vi "test_F9P.vi"() -> ()   [LabVIEW 2019] (continued)
N,3.578,K,A*10\r\n$GNGGA,064213.00,3723.60796,N,12656.94619,E,1,12,0.68,49.8,M,18.5,M,,*7A\r\n$GNGSA,A,3,17,19,06,05,02,12,09,,,,,,1.13,0.68,0.90,1*00\r\n$GNGSA,A,3,85,70,71,72,,,,,,,,,1.13,0.68,0.90,2*0F\r\n$GNGSA,A,3,36,19,11,04,09,12,,,,,,,1.13,0.68,0.90,3*04\r\n$GNGSA,A,3,28,14,13,11,33,08,10,,,,,,1.13,0.68,0.90,4*04\r\n$GPGSV,4,1,13,02,65,334,34,04,08,037,26,05,48,261,38,06,58,076,46,1*62\r\n$GPGSV,4,2,13,07,06,105,,09,38,057,36,12,18,263,26,13,08,191,,1*6A\r\n$GPGSV,4,3,13,17,19,158,28,19,37,161,30,25,11,294,20,29,07,323,10,1*65\r\n$GPGSV,4,4,13,30,01,134,,1*52\r\n$GPGSV,4,1,13,02,65,334,,04,08,037,19,05,48,261,37,06,58,076,31,6*61\r\n$GPGSV,4,2,13,07,06,105,,09,38,057,33,12,18,263,21,13,08,191,,6*6F\r\n$GPGSV,4,3,13,17,19,158,20,19,37,161,,25,11,294,16,29,07,323,,6*6D\r\n$GPGSV,4,4,13,30,01,134,,6*55\r\n$GLGSV,2,1,06,70,55,030,32,71,68,223,43,72,17,216,27,84,09,133,11,1*73\r\n$GLGSV,2,2,06,85,63,111,32,86,51,337,,1*7B\r\n$GLGSV,2,1,06,70,55,030,,71,68,223,34,72,17,216,20,84,09,133,11,3*77\r\n$GLGSV,2,2,06,85,63,111,25,86,51,337,,3*7F\r\n$GAGSV,3,1,09,02,04,288,08,04,68,087,43,09,44,196,29,11,77,034,39,7*77\r\n$GAGSV,3,2,09,12,32,114,28,18,55,286,44,19,17,042,25,25,01,241,,7*7C\r\n$GAGSV,3,3,09,36,34,314,20,7*4C\r\n$GAGSV,3,1,09,02,04,288,,04,68,087,36,09,44,196,24,11,77,034,26,2*7B\r\n$GAGSV,3,2,09,12,32,114,22,18,55,286,41,19,17,042,23,25,01,241,,2*70\r\n$GAGSV,3,3,09,36,34,314,21,2*48\r\n$GBGSV,4,1,13,04,35,133,,05,09,257,,06,27,182,,07,09,201,,1*7B\r\n$GBGSV,4,2,13,08,65,355,26,09,07,194,,10,16,222,,11,38,142,27,1*71\r\n$GBGSV,4,3,13,13,50,314,19,14,77,038,42,28,58,310,30,33,72,237,42,1*71\r\n$GBGSV,4,4,13,34,13,141,,1*45\r\n$GBGSV,4,1,13,04,35,133,,05,09,257,,06,27,182,,07,09,201,,3*79\r\n$GBGSV,4,2,13,08,65,355,26,09,07,194,,10,16,222,19,11,38,142,29,3*75\r\n$GBGSV,4,3,13,13,50,314,19,14,77,038,38,28,58,310,,33,72,237,,3*7B\r\n$GBGSV,4,4,13,34,13,141,,3*47\r\n$GNGLL,3723.60796,N,12656.94619,E,064213.00,A,A*7B\r\n$GNRMC,064214.00,A,3723.60817,N,12656.94692,E,2.319,73.22,250720,,,A,V*3B\r\n$GNVTG,73.22,T,,M,2.319,N,4.294,K,A*15\r\n$GNGGA,064214.00,3723.60817,N,12656.94692,E,1,12,0.71,49.3,M,18.5,M,,*7B\r\n$GNGSA,A,3,17,19,06,05,02,12,09,,,,,,1.14,0.71,0.90,1*0F\r\n$GNGSA,A,3,85,70,71,72,,,,,,,,,1.14,0.71,0.90,2*00\r\n$GNGSA,A,3,36,19,11,04,09,12,,,,,,,1.14,0.71,0.90,3*0B\r\n$GNGSA,A,3,28,14,13,11,33,08,10,,,,,,1.14,0.71,0.90,4*0B\r\n$GPGSV,4,1,13,02,65,334,29,04,08,037,31,05,48,261,39,06,58,076,39,1*61\r\n$GPGSV,4,2,13,07,06,105,,09,38,057,39,12,18,263,29,13,08,191,,1*6A\r\n$GPGSV,4,3,13,17,19,158,27,19,37,161,36,25,11,294,20,29,07,323,08,1*65\r\n$GPGSV,4,4,13,30,01,134,,1*52\r\n$GPGSV,4,1,13,02,65,334,,04,08,037,21,05,48,261,37,06,58,076,34,6*6F\r\n$GPGSV,4,2,13,07,06,105,,09,38,057,32,12,18,263,21,13,08,191,,6*6E\r\n$GPGSV,4,3,13,17,19,158,20,19,37,161,,25,11,294,14,29,07,323,,6*6F\r\n$GPGSV,4,4,13,30,01,134,,6*55\r\n$GLGSV,2,1,06,70,55,030,31,71,68,223,38,72,17,216,31,84,09,133,08,1*73\r\n$GLGSV,2,2,06,85,63,111,32,86,51,337,,1*7B\r\n$GLGSV,2,1,06,70,55,030,,71,68,223,29,72,17,216,21,84,09,133,12,3*79\r\n$GLGSV,2,2,06,85,63,111,22,86,51,337,,3*78\r\n$GAGSV,3,1,09,02,04,288,10,04,68,087,44,09,44,196,29,11,77,034,35,7*75\r\n$GAGSV,3,2,09,12,32,114,23,18,55,286,33,19,17,042,31,25,01,241,,7*72\r\n$GAGSV,3,3,09,36,34,314,21,7*4D\r\n$GAGSV,3,1,09,02,04,288,,04,68,087,35,09,44,196,22,11,77,034,31,2*78\r\n$GAGSV,3,2,09,12,32,114,21,18,55,286,42,19,17,042,23,25,01,241,,2*70\r\n$GAGSV,3,3,09,36,34,314,21,2*48\r\n$GBGSV,4,1,13,04,35,133,,05,09,257,,06,27,182,,07,09,201,,1*7B\r\n$GBGSV,4,2,13,08,65,355,31,09,07,194,,10,16,222,,11,38,142,19,1*7A\r\n$GBGSV,4,3,13,13,50,314,19,14,77,038,39,28,58,310,34,33,72,237,36,1*7A\r\n$GBGSV,4,4,13,34,13,141,,1*45\r\n$GBGSV,4,1,13,04,35,133,,05,09,257,,06,27,182,,07,09,201,,3*79\r\n$GBGSV,4,2,13,08,65,355,31,09,07,194,,10,16,222,19,11,38,142,24,3*7E\r\n$GBGSV,4,3,13,13,50,314,19,14,77,038,29,28,58,310,,33,72,237,,3*7B\r\n$GBGSV,4,4,13,34,13,141,,3*47\r\n$GNGLL,3723.60817,N,12656.94692,E,064214.00,A,A*79\r\n$GNRMC,064215.00,A,3723.60846,N,12656.94770,E,2.329,70.21,250720,,,A,V*30\r\n$GNVTG,70.21,T,,M,2.329,N,4.313,K,A*18\r\n$GNGGA,064215.00,3723.60846,N,12656.94770,E,1,12,0.73,48.8,M,18.5,M,,*7B\r\n$GNGSA,A,3,17,19,06,05,02,12,09,,,,,,1.16,0.73,0.90,1*0F\r\n$GNGSA,A,3,85,70,71,72,,,,,,,,,1.16,0.73,0.90,2*00\r\n$GNGSA,A,3,36,19,11,04,09,12,,,,,,,1.16,0.73,0.90,3*0B\r\n$GNGSA,A,3,28,14,13,11,33,08,10,,,,,,1.16,0.73,0.90,4*0B\r\n$GPGSV,4,1,13,02,65,334,33,04,08,037,31,05,48,261,40,06,58,076,43,1*69\r\n$GPGSV,4,2,13,07,06,105,,09,38,057,40,12,18,263,30,13,08,191,,1*6C\r\n$GPGSV,4,3,13,17,19,158,26,19,37,161,32,25,11,294,19,29,07,323,08,1*6A\r\n$GPGSV,4,4,13,30,01,134,,1*52\r\n$GPGSV,4,1,13,02,65,334,,04,08,037,22,05,48,261,36,06,58,076,34,6*6D\r\n$GPGSV,4,2,13,07,06,105,,09,38,057,35,12,18,263,20,13,08,191,,6*68\r\n$GPGSV,4,3,13,17,19,158,19,19,37,161,,25,11,294,12,29,07,323,,6*63\r\n$GPGSV,4,4,13,30,01,134,,6*55\r\n$GLGSV,2,1,06,70,55,030,35,71,68,223,38,72,17,216,21,84,09,133,10,1*7F\r\n$GLGSV,2,2,06,85,63,111,36,86,51,337,,1*7F\r\n$GLGSV,2,1,06,70,55,030,,71,68,223,28,72,17,216,18,84,09,133,12,3*72\r\n$GLGSV,2,2,06,85,63,111,24,86,51,337,,3*7E\r\n$GAGSV,3,1,09,02,04,287,07,04,68,087,41,09,44,196,29,11,77,034,37,7*7B\r\n$GAGSV,3,2,09,12,32,114,29,18,55,286,32,19,17,042,26,25,01,241,,7*7F\r\n$GAGSV,3,3,09,36,34,314,22,7*4E\r\n$GAGSV,3,1,09,02,04,287,,04,68,087,36,09,44,196,24,11,77,034,30,2*73\r\n$GAGSV,3,2,09,12,32,114,19,18,55,286,42,19,17,042,29,25,01,241,,2*71\r\n$GAGSV,3,3,09,36,34,314,20,2*49\r\n$GBGSV,4,1,13,04,35,133,,05,09,257,,06,27,182,,07,09,201,,1*7B\r\n$GBGSV,4,2,13,08,65,355,35,09,07,194,,10,16,222,18,11,38,142,32,1*7E\r\n$GBGSV,4,3,13,13,50,314,20,14,77,038,41,28,58,310,31,33,72,237,39,1*75\r\n$GBGSV,4,4,13,34,13,141,,1*45\r\n$GBGSV,4,1,13,04,35,133,,05,09,257,,06,27,182,,07,09,201,,3*79\r\n$GBGSV,4,2,13,08,65,355,25,09,07,194,,10,16,222,19,11,38,142,36,3*78\r\n$GBGSV,4,3,13,13,50,314,20,14,77,038,38,28,58,310,,33,72,237,,3*71\r\n$GBGSV,4,4,13,34,13,141,,3*47\r\n$GNGLL,3723.60846,N,12656.94770,E,064215.00,A,A*71\r\n$GNRMC,064216.00,A,3723.60894,N,12656.94830,E,2.005,64.28,250720,,,A,V*36\r\n$GNVTG,64.28,T,,M,2.005,N,3.713,K,A*1A\r\n$GNGGA,064216.00,3723.60894,N,12656.94830,E,1,12,0.68,47.9,M,18.5,M,,*78\r\n$GNGSA,A,3,17,19,06,05,02,12,09,,,,,,1.13,0.68,0.90,1*00\r\n$GNGSA,A,3,85,70,71,72,,,,,,,,,1.13,0.68,0.90,2*0F\r\n$GNGSA,A,3,36,19,11,04,09,12,,,,,,,1.13,0.68,0.90,3*04\r\n$GNGSA,A,3,28,14,13,11,33,08,10,,,,,,1.13,0.68,0.90,4*04\r\n$GPGSV,4,1,13,02,65,334,28,04,08,037,24,05,48,261,40,06,58,076,46,1*62\r\n$GPGSV,4,2,13,07,06,105,,09,38,057,40,12,18,263,25,13,08,191,,1*68\r\n$GPGSV,4,3,13,17,19,158,26,19,37,161,35,25,11,294,20,29,07,323,09,1*66\r\n$GPGSV,4,4,13,30,01,134,,1*52\r\n$GPGSV,4,1,13,02,65,334,,04,08,037,20,05,48,261,31,06,58,076,33,6*6F\r\n$GPGSV,4,2,13,07,06,105,,09,38,057,35,12,18,263,18,13,08,191,,6*63\r\n$GPGSV,4,3,13,17,19,158,17,19,37,161,,25,11,294,10,29,07,323,,6*6F\r\n$GPGSV,4,4,13,30,01,134,,6*55\r\n$GLGSV,2,1,06,70,55,030,36,71,68,223,40,72,17,216,23,84,09,133,10,1*71\r\n$GLGSV,2,2,06,85,63,111,32,86,51,337,,1*7B\r\n$GLGSV,2,1,06,70,55,030,,71,68,223,26,72,17,216,18,84,09,133,09,3*76\r\n$GLGSV,2,2,06,85,63,111,24,86,51,337,,3*7E\r\n$GAGSV,3,1,09,02,04,287,08,04,68,087,42,09,44,196,34,11,77,034,35,7*79\r\n$GAGSV,3,2,09,12,32,114,25,18,55,286,32,19,17,042,28,25,01,241,,7*7D\r\n$GAGSV,3,3,09,36,34,314,22,7*4E\r\n$GAGSV,3,1,09,02,04,287,,04,68,087,30,09,44,196,24,11,77,034,25,2*71\r\n$GAGSV,3,2,09,12,32,114,20,18,55,286,35,19,17,042,22,25,01,241,,2*70\r\n$GAGSV,3,3,09,36,34,314,21,2*48\r\n$GBGSV,4,1,13,04,35,133,,05,09,257,,06,27,182,,07,09,201,,1*7B\r\n$GBGSV,4,2,13,08,65,355,26,09,07,194,,10,16,222,19,11,38,142,28,1*76\r\n$GBGSV,4,3,13,13,50,314,19,14,77,038,40,28,58,310,31,33,72,237,36,1*71\r\n$GBGSV,4,4,13,34,13,141,,1*45\r\n$GBGSV,4,1,13,04,35,133,,05,09,257,,06,27,182,,07,09,201,,3*79\r\n$GBGSV,4,2,13,08,65,355,26,09,07,194,,10,16,222,18,11,38,142,19,3*77\r\n$GBGSV,4,3,13,13,50,314,18,14,77,038,24,28,58,310,,33,72,237,,3*77\r\n$GBGSV,4,4,13,34,13,141,,3*47\r\n$GNGLL,3723.60894,N,12656.94830,E,064216.00,A,A*76\r\n$GNRMC,064217.00,A,3723.60911,N,12656.94907,E,2.470,76.30,250720,,,A,V*32\r\n$GNVTG,76.30,T,,M,2.470,N,4.575,K,A*13\r\n$GNGGA,064217.00,3723.60911,N,12656.94907,E,1,12,0.73,47.4,M,18.5,M,,*77\r\n$GNGSA,A,3,17,19,06,05,02,12,09,,,,,,1.16,0.73,0.90,1*0F\r\n$GNGSA,A,3,85,70,71,72,,,,,,,,,1.16,0.73,0.90,2*00\r\n$GNGSA,A,3,36,19,11,04,09,12,,,,,,,1.16,0.73,0.90,3*0B\r\n$GNGSA,A,3,28,14,13,11,33,08,10,,,,,,1.16,0.73,0.90,4*0B\r\n$GPGSV,4,1,13,02,65,334,32,04,08,037,25,05,48,261,38,06,58,076,47,1*66\r\n$GPGSV,4,2,13,07,06,105,,09,38,057,40,12,18,263,31,13,08,191,,1*6D\r\n$GPGSV,4,3,13,17,19,158,25,19,37,161,28,25,11,294,20,29,07,323,10,1*61\r\n$GPGSV,4,4,13,30,01,134,,1*52\r\n$GPGSV,4,1,13,02,65,334,,04,08,037,20,05,48,261,31,06,58,076,34,6*68\r\n$GPGSV,4,2,13,07,06,105,,09,38,057,32,12,18,263,15,13,08,191,,6*69\r\n$GPGSV,4,3,13,17,19,158,15,19,37,161,,25,11,294,08,29,07,323,,6*64\r\n$GPGSV,4,4,13,30,01,134,,6*55\r\n$GLGSV,2,1,06,70,55,030,36,71,68,223,33,72,17,216,24,84,09,133,08,1*7B\r\n$GLGSV,2,2,06,85,63,111,32,86,51,337,,1*7B\r\n$GLGSV,2,1,06,70,55,030,,71,68,223,25,72,17,216,18,84,09,133,06,3*7A\r\n$GLGSV,2,2,06,85,63,111,30,86,51,337,,3*7B\r\n$GAGSV,3,1,09,02,04,287,11,04,68,085,43,09,44,196,29,11,77,034,37,7*7C\r\n$GAGSV,3,2,09,12,32,114,27,18,55,286,36,19,17,042,29,25,01,241,,7*7A\r\n$GAGSV,3,3,09,36,34,314,22,7*4E\r\n$GAGSV,3,1,09,02,04,287,,04,68,085,33,09,44,196,24,11,77,034,31,2*75\r\n$GAGSV,3,2,09,12,32,114,18,18,55,286,39,19,17,042,22,25,01,241,,2*77\r\n$GAGSV,3,3,09,36,34,314,20,2*49\r\n$GBGSV,4,1,13,04,35,133,,05,09,257,,06,27,182,,07,09,201,,1*7B\r\n$GBGSV,4,2,13,08,65,355,30,09,07,194,,10,16,222,19,11,38,142,25,1*7C\r\n$GBGSV,4,3,13,13,50,314,21,14,77,038,37,28,58,310,26,33,72,237,39,1*73\r\n$GBGSV,4,4,13,34,13,141,,1*45\r\n$GBGSV,4,1,13,04,35,133,,05,09,257,,06,27,182,,07,09,201,,3*79\r\n$GBGSV,4,2,13,08,65,355,26,09,07,194,,10,16,222,16,11,38,142,27,3*74\r\n$GBGSV,4,3,13,13,50,314,18,14,77,038,34,28,58,310,,33,72,237,,3*76\r\n$GBGSV,4,4,13,34,13,141,,3*47\r\n$GNGLL,3723.60911,N,12656.94907,E,064217.00,A,A*7E\r\n$GNRMC,064218.00,A,3723.60947,N,12656.94982,E,2.502,67.45,250720,,,A,V*35\r\n$GNVTG,67.45,T,,M,2.502,N,4.634,K,A*13\r\n$GNGGA,064218.00,3723.60947,N,12656.94982,E,1,12,0.70,47.0,M,18.5,M,,*71\r\n$GNGSA,A,3,17,19,06,05,02,12,09,,,,,,1.14,0.70,0.90,1*0E\r\n$GNGSA,A,3,85,70,71,72,,,,,,,,,1.14,0.70,0.90,2*01\r\n$GNGSA,A,3,36,19,11,04,09,12,,,,,,,1.14,0.70,0.90,3*0A\r\n$GNGSA,A,3,28,14,13,11,33,08,10,,,,,,1.14,0.70,0.90,4*0A\r\n$GPGSV,4,1,13,02,65,334,28,04,08,037,24,05,48,261,39,06,58,076,49,1*63\r\n$GPGSV,4,2,13,07,06,105,,09,38,057,40,12,18,263,31,13,08,191,,1*6D\r\n$GPGSV,4,3,13,17,19,158,25,19,37,161,27,25,11,294,20,29,07,323,09,1*66\r\n$GPGSV,4,4,13,30,01,134,,1*52\r\n$GPGSV,4,1,13,02,65,334,,04,08,037,18,05,48,261,32,06,58,076,30,6*64\r\n$GPGSV,4,2,13,07,06,105,,09,38,057,33,12,18,263,14,13,08,191,,6*69\r\n$GPGSV,4,3,13,17,19,158,14,19,37,161,,25,11,294,07,29,07,323,,6*6A\r\n$GPGSV,4,4,13,30,01,134,,6*55\r\n$GLGSV,2,1,06,70,55,030,34,71,68,223,38,72,17,216,25,84,09,133,10,1*7A\r\n$GLGSV,2,2,06,85,63,111,39,86,51,337,,1*70\r\n$GLGSV,2,1,06,70,55,030,,71,68,223,31,72,17,216,18,84,09,133,10,3*78\r\n$GLGSV,2,2,06,85,63,111,25,86,51,337,,3*7F\r\n$GAGSV,3,1,09,02,04,287,10,04,68,085,42,09,44,196,28,11,77,034,37,7*7D\r\n$GAGSV,3,2,09,12,32,114,26,18,55,286,37,19,17,042,28,25,01,241,,7*7B\r\n$GAGSV,3,3,09,36,34,314,23,7*4F\r\n$GAGSV,3,1,09,02,04,287,,04,68,085,33,09,44,196,23,11,77,034,30,2*73\r\n$GAGSV,3,2,09,12,32,114,17,18,55,286,43,19,17,042,21,25,01,241,,2*76\r\n$GAGSV,3,3,09,36,34,314,19,2*43\r\n$GBGSV,4,1,13,04,35,133,,05,09,257,,06,27,182,,07,09,201,25,1*7C\r\n$GBGSV,4,2,13,08,65,355,27,09,07,194,,10,16,222,19,11,38,142,32,1*7C\r\n$GBGSV,4,3,13,13,50,314,20,14,77,038,42,28,58,310,28,33,72,237,36,1*71\r\n$GBGSV,4,4,13,34,13,141,,1*45\r\n$GBGSV,4,1,13,04,35,133,,05,09,257,,06,27,182,,07,09,201,,3*79\r\n$GBGSV,4,2,13,08,65,355,28,09,07,194,,10,16,222,16,11,38,142,20,3*7D\r\n$GBGSV,4,3,13,13,50,314,,14,77,038,35,28,58,310,,33,72,237,,3*7E\r\n$GBGSV,4,4,13,34,13,141,,3*47\r\n$GNGLL,3723.60947,N,12656.94982,E,064218.00,A,A*7F\r\n$GNRMC,064219.00,A,3723.60983,N,12656.95051,E,2.178,73.49,250720,,,A,V*3A\r\n$GNVTG,73.49,T,,M,2.178,N,4.034,K,A*15\r\n$GNGGA,064219.00,3723.60983,N,12656.95051,E,1,12,0.70,47.2,M,18.5,M,,*7C\r\n$GNGSA,A,3,17,19,06,05,02,12,09,,,,,,1.14,0.70,0.90,1*0E\r\n$GNGSA,A,3,85,70,71,72,,,,,,,,,1.14,0.70,0.90,2*01\r\n$GNGSA,A,3,36,19,11,04,09,12,,,,,,,1.14,0.70,0.90,3*0A\r\n$GNGSA,A,3,28,14,13,11,33,08,10,,,,,,1.14,0.70,0.90,4*0A\r\n$GPGSV,4,1,13,02,65,334,27,04,08,037,30,05,48,261,39,06,58,076,45,1*65\r\n$GPGSV,4,2,13,07,06,105,,09,38,057,44,12,18,263,26,13,08,191,,1*6F\r\n$GPGSV,4,3,13,17,19,158,24,19,37,161,28,25,11,294,19,29,07,323,08,1*63\r\n$GPGSV,4,4,13,30,01,134,,1*52\r\n$GPGSV,4,1,13,02,65,334,,04,08,037,21,05,48,261,36,06,58,076,34,6*6E\r\n$GPGSV,4,2,13,07,06,105,,09,38,057,36,12,18,263,14,13,08,191,,6*6C\r\n$GPGSV,4,3,13,17,19,158,14,19,37,161,,25,11,294,,29,07,323,,6*6D\r\n$GPGSV,4,4,13,30,01,134,,6*55\r\n$GLGSV,2,1,06,70,55,030,29,71,68,223,38,72,17,216,31,84,09,133,10,1*73\r\n$GLGSV,2,2,06,85,63,111,35,86,51,337,,1*7C\r\n$GLGSV,2,1,06,70,55,030,,71,68,223,26,72,17,216,19,84,09,133,11,3*7E\r\n$GLGSV,2,2,06,85,63,111,26,86,51,337,,3*7C\r\n$GAGSV,3,1,09,02,04,287,09,04,68,085,39,09,44,196,27,11,77,034,38,7*79\r\n$GAGSV,3,2,09,12,32,114,27,18,55,286,35,19,17,042,29,25,01,241,,7*79\r\n$GAGSV,3,3,09,36,34,314,23,7*4F\r\n$GAGSV,3,1,09,02,04,287,,04,68,085,38,09,44,196,29,11,77,034,31,2*73\r\n$GAGSV,3,2,09,12,32,114,18,18,55,286,42,19,17,042,29,25,01,241,,2*70\r\n$GAGSV,3,3,09,36,34,314,21,2*48\r\n$GBGSV,4,1,13,04,35,133,,05,09,257,,06,27,182,,07,09,201,21,1*78\r\n$GBGSV,4,2,13,08,65,355,35,09,07,194,,10,16,222,19,11,38,142,32,1*7F\r\n$GBGSV,4,3,13,13,50,314,19,14,77,038,41,28,58,310,26,33,72,237,40,1*77\r\n$GBGSV,4,4,13,34,13,141,,1*45\r\n$GBGSV,4,1,13,04,35,133,,05,09,257,,06,27,182,,07,09,201,,3*79\r\n$GBGSV,4,2,13,08,65,355,33,09,07,194,,10,16,222,19,11,38,142,24,3*7C\r\n$GBGSV,4,3,13,13,50,314,23,14,77,038,41,28,58,310,,33,72,237,,3*7C\r\n$GBGSV,4,4,13,34,13,141,,3*47\r\n$GNGLL,3723.60983,N,12656.95051,E,064219.00,A,A*70\r\n$GNRMC,064220.00,A,3723.61003,N,12656.95147,E,2.836,76.56,250720,,,A,V*3E\r\n$GNVTG,76.56,T,,M,2.836,N,5.252,K,A*1E\r\n$GNGGA,064220.00,3723.61003,N,12656.95147,E,1,12,0.71,47.0,M,18.5,M,,*73\r\n$GNGSA,A,3,17,19,06,05,02,12,09,,,,,,1.14,0.71,0.90,1*0F\r\n$GNGSA,A,3,85,70,71,72,,,,,,,,,1.14,0.71,0.90,2*00\r\n$GNGSA,A,3,36,19,11,04,09,12,,,,,,,1.14,0.71,0.90,3*0B\r\n$GNGSA,A,3,28,14,13,11,33,08,10,,,,,,1.14,0.71,0.90,4*0B\r\n$GPGSV,4,1,13,02,65,334,35,04,08,037,29,05,48,261,38,06,58,076,49,1*63\r\n$GPGSV,4,2,13,07,06,105,,09,38,057,39,12,18,263,26,13,08,191,,1*65\r\n$GPGSV,4,3,13,17,19,158,23,19,37,161,21,25,11,294,18,29,07,323,08,1*6C\r\n$GPGSV,4,4,13,30,01,134,,1*52\r\n$GPGSV,4,1,13,02,65,334,,04,08,037,21,05,48,261,33,06,58,076,31,6*6E\r\n$GPGSV,4,2,13,07,06,105,,09,38,057,37,12,18,263,13,13,08,191,,6*6A\r\n$GPGSV,4,3,13,17,19,158,12,19,37,161,,25,11,294,,29,07,323,,6*6B\r\n$GPGSV,4,4,13,30,01,134,,6*55\r\n$GLGSV,2,1,06,70,55,030,30,71,68,223,36,72,17,216,27,84,09,133,11,1*73\r\n$GLGSV,2,2,06,85,63,111,34,86,51,337,,1*7D\r\n$GLGSV,2,1,06,70,55,030,,71,68,223,27,72,17,216,20,84,09,133,11,3*75\r\n$GLGSV,2,2,06,85,63,111,26,86,51,337,,3*7C\r\n$GAGSV,3,1,09,02,04,287,10,04,68,085,40,09,44,196,32,11,77,034,38,7*7B\r\n$GAGSV,3,2,09,12,32,114,33,18,55,286,38,19,17,042,29,25,01,241,,7*71\r\n$GAGSV,3,3,09,36,34,314,22,7*4E\r\n$GAGSV,3,1,09,02,04,287,,04,68,085,37,09,44,196,29,11,77,034,34,2*79\r\n$GAGSV,3,2,09,12,32,114,29,18,55,286,31,19,17,042,28,25,01,241,,2*77\r\n$GAGSV,3,3,09,36,34,314,21,2*48\r\n$GBGSV,4,1,13,04,35,133,,05,09,257,,06,27,182,,07,09,201,19,1*73\r\n$GBGSV,4,2,13,08,65,355,36,09,07,194,,10,16,222,19,11,38,142,25,1*7A\r\n$GBGSV,4,3,13,13,50,314,19,14,77,038,40,28,58,310,14,33,72,237,35,1*75\r\n$GBGSV,4,4,13,34,13,141,,1*45\r\n$GBGSV,4,1,13,04,35,133,,05,09,257,,06,27,182,,07,09,201,,3*79\r\n$GBGSV,4,2,13,08,65,355,33,09,07,194,,10,16,222,21,11,38,142,25,3*76\r\n$GBGSV,4,3,13,13,50,314,20,14,77,038,36,28,58,310,,33,72,237,,3*7F\r\n$GBGSV,4,4,13,34,13,141,,3*47\r\n$GNGLL,3723.61003,N,12656.95147,E,064220.00,A,A*7C\r\n$GNRMC,064221.00,A,3723.61019,N,12656.95243,E,2.402,71.98,250720,,,A,V*3D\r\n$GNVTG,71.98,T,,M,2.402,N,4.448,K,A*1C\r\n$GNGGA,064221.00,3723.61019,N,12656.95243,E,1,12,0.70,46.6,M,18.5,M,,*78\r\n$GNGSA,A,3,17,19,06,05,02,12,09,,,,,,1.14,0.70,0.90,1*0E\r\n$GNGSA,A,3,85,70,71,72,,,,,,,,,1.14,0.70,0.90,2*01\r\n$GNGSA,A,3,36,19,11,04,09,12,,,,,,,1.14,0.70,0.90,3*0A\r\n$GNGSA,A,3,28,14,13,11,33,08,10,,,,,,1.14,0.70,0.90,4*0A\r\n$GPGSV,4,1,13,02,65,334,39,04,08,037,34,05,48,261,38,06,58,076,40,1*6A\r\n$GPGSV,4,2,13,07,06,105,,09,38,057,40,12,18,263,27,13,08,191,,1*6A\r\n$GPGSV,4,3,13,17,19,158,23,19,37,161,36,25,11,294,18,29,07,323,08,1*6A\r\n$GPGSV,4,4,13,30,01,134,,1*52\r\n$GPGSV,4,1,13,02,65,334,,04,08,037,21,05,48,261,33,06,58,076,32,6*6D\r\n$GPGSV,4,2,13,07,06,105,,09,38,057,37,12,18,263,14,13,08,191,,6*6D\r\n$GPGSV,4,3,13,17,19,158,13,19,37,161,,25,11,294,,29,07,323,,6*6A\r\n$GPGSV,4,4,13,30,01,134,,6*55\r\n$GLGSV,2,1,06,70,55,030,31,71,68,223,42,72,17,216,27,84,09,133,12,1*72\r\n$GLGSV,2,2,06,85,63,111,32,86,51,337,,1*7B\r\n$GLGSV,2,1,06,70,55,030,,71,68,223,27,72,17,216,20,84,09,133,09,3*7C\r\n$GLGSV,2,2,06,85,63,111,27,86,51,337,,3*7D\r\n$GAGSV,3,1,09,02,04,287,09,04,68,085,38,09,44,196,29,11,77,034,38,7*76\r\n$GAGSV,3,2,09,12,32,114,27,18,55,286,33,19,17,042,19,25,01,241,,7*7C\r\n$GAGSV,3,3,09,36,34,314,22,7*4E\r\n$GAGSV,3,1,09,02,04,287,,04,68,085,34,09,44,196,27,11,77,034,34,2*74\r\n$GAGSV,3,2,09,12,32,114,,18,55,286,37,19,17,042,28,25,01,241,,2*7A\r\n$GAGSV,3,3,09,36,34,314,21,2*48\r\n$GBGSV,4,1,13,04,35,133,,05,09,257,,06,27,182,,07,09,201,19,1*73\r\n$GBGSV,4,2,13,08,65,355,40,09,07,194,,10,16,222,18,11,38,142,25,1*7A\r\n$GBGSV,4,3,13,13,50,314,18,14,77,038,38,28,58,310,28,33,72,237,36,1*77\r\n$GBGSV,4,4,13,34,13,141,,1*45\r\n$GBGSV,4,1,13,04,35,133,,05,09,257,,06,27,182,,07,09,201,,3*79\r\n$GBGSV,4,2,13,08,65,355,36,09,07,194,,10,16,222,19,11,38,142,27,3*7A\r\n$GBGSV,4,3,13,13,50,314,,14,77,038,36,28,58,310,,33,72,237,,3*7D\r\n$GBGSV,4,4,13,34,13,141,,3*47\r\n$GNGLL,3723.61019,N,12656.95243,E,064221.00,A,A*71\r\n$GNRMC,064222.00,A,3723.61077,N,12656.95320,E,2.416,69.88,250720,,,A,V*3F\r\n$GNVTG,69.88,T,,M,2.416,N,4.474,K,A*1E\r\n$GNGGA,064222.00,3723.61077,N,12656.95320,E,1,12,0.68,46.9,M,18.5,M,,*71\r\n$GNGSA,A,3,17,19,06,05,02,12,09,,,,,,1.13,0.68,0.90,1*00\r\n$GNGSA,A,3,85,70,71,72,,,,,,,,,1.13,0.68,0.90,2*0F\r\n$GNGSA,A,3,36,19,11,04,09,12,,,,,,,1.13,0.68,0.90,3*04\r\n$GNGSA,A,3,28,14,13,11,33,08,10,,,,,,1.13,0.68,0.90,4*04\r\n$GPGSV,4,1,13,02,65,334,35,04,08,037,31,05,48,261,35,06,58,076,39,1*60\r\n$GPGSV,4,2,13,07,06,105,,09,38,057,46,12,18,263,25,13,08,191,,1*6E\r\n$GPGSV,4,3,13,17,19,158,24,19,37,161,37,25,11,294,18,29,07,323,07,1*63\r\n$GPGSV,4,4,13,30,01,134,,1*52\r\n$GPGSV,4,1,13,02,65,334,,04,08,037,22,05,48,261,28,06,58,076,28,6*6F\r\n$GPGSV,4,2,13,07,06,105,,09,38,057,39,12,18,263,14,13,08,191,,6*63\r\n$GPGSV,4,3,13,17,19,158,15,19,37,161,,25,11,294,,29,07,323,,6*6C\r\n$GPGSV,4,4,13,30,01,134,,6*55\r\n$GLGSV,2,1,06,70,55,030,34,71,68,223,40,72,17,216,32,84,09,133,09,1*7B\r\n$GLGSV,2,2,06,85,63,111,32,86,51,337,,1*7B\r\n$GLGSV,2,1,06,70,55,030,,71,68,223,28,72,17,216,20,84,09,133,10,3*7B\r\n$GLGSV,2,2,06,85,63,111,25,86,51,337,,3*7F\r\n$GAGSV,3,1,09,02,04,287,08,04,68,085,39,09,44,196,30,11,78,037,35,7*7F\r\n$GAGSV,3,2,09,12,32,114,27,18,55,286,36,19,17,042,28,25,01,241,,7*7B\r\n$GAGSV,3,3,09,36,34,314,21,7*4D\r\n$GAGSV,3,1,09,02,04,287,,04,68,085,34,09,44,196,25,11,78,037,33,2*7D\r\n$GAGSV,3,2,09,12,32,114,27,18,55,286,43,19,17,042,28,25,01,241,,2*7C\r\n$GAGSV,3,3,09,36,34,314,21,2*48\r\n$GBGSV,4,1,13,04,35,133,,05,09,257,,06,
